vi "实验5 相移键控TX.vi"() -> ()   [LabVIEW 2015]
uses:
  SubVI/SubVI TX Channel Model Params.ctl
  SubVI/SubVI TX HW Aprams.ctl
  <instrlib>/niUSRP/niUSRP Write Tx Data (CDB Cluster).vi
panel:
  out "发送时间":dbl format="%#_4ps"
  out "码元数据量":i32
  in  "设置选项卡":enum32{"硬件设置", "信道设置", "调制设置", "调试显示"}(tab)
  in  "硬件设置":T1={"设备IP地址"="192.168.10.2", "天线"="TX1", "载波频率 (Hz)"=800000000.0, "增益 (dB)"=10.0} {"增益 (dB)" format="%.2f"; "载波频率 (Hz)" format="%.2p"}
  in  "信道模型":T2={"信道模型"="AWGN", "噪声能量 (dB)"=-100.0, "信道响应"=[], "频偏 "=0.0, "延迟 (秒)"=0.0}
  in  "调制设置":T3={"调制方式"="QPSK", "脉冲成形参数 "={"调制方式 "=enum."PSK", "脉冲成形滤波器 "=enum."根升余弦", "滤波器参数"=0.5, "滤波长度 (码元)"=8}, "TX 过采样因子"=4, "TX 采样率"=500000.0} {"TX 采样率" items=["25M"=25000000.0, "20M"=20000000.0, "16.6667M"=16666666.666667, "14.2857M"=14285714.285714, "12.5M"=12500000.0, "11.1111M"=11111111.111111, "10M"=10000000.0, "9.09091M"=9090909.090909, "8.33333M"=8333333.333333, "7.69231M"=7692307.692308, "7.14286M"=7142857.142857, "6.66667M"=6666666.666667, "6.25M"=6250000.0, "5.88235M"=5882352.941176, "5.55556M"=5555555.555556, "5.26316M"=5263157.894737, "5M"=5000000.0, "4.7619M"=4761904.761905, "4.54545M"=4545454.545455, "4.34783M"=4347826.086957, "4.16667M"=4166666.666667, "4M"=4000000.0, "3.84615M"=3846153.846154, "3.7037M"=3703703.703704, "3.57143M"=3571428.571429, "3.44828M"=3448275.862069, "3.33333M"=3333333.333333, "3.22581M"=3225806.451613, "3.125M"=3125000.0, "3.0303M"=3030303.030303, "2.94118M"=2941176.470588, "2.85714M"=2857142.857143, "2.77778M"=2777777.777778, "2.7027M"=2702702.702703, "2.63158M"=2631578.947368, "2.5641M"=2564102.564103, "2.5M"=2500000.0, "2.43902M"=2439024.390244, "2.38095M"=2380952.380952, "2.32558M"=2325581.395349, "2.27273M"=2272727.272727, "2.22222M"=2222222.222222, "2.17391M"=2173913.043478, "2.12766M"=2127659.574468, "2.08333M"=2083333.333333, "2.04082M"=2040816.326531, "2M"=2000000.0, "1.96078M"=1960784.313725, "1.92308M"=1923076.923077, "1.88679M"=1886792.45283, "1.85185M"=1851851.851852, "1.81818M"=1818181.818182, "1.78571M"=1785714.285714, "1.75439M"=1754385.964912, "1.72414M"=1724137.931034, "1.69492M"=1694915.254237, "1.66667M"=1666666.666667, "1.63934M"=1639344.262295, "1.6129M"=1612903.225806, "1.5873M"=1587301.587302, "1.5625M"=1562500.0, "1.53846M"=1538461.538462, "1.51515M"=1515151.515152, "1.49254M"=1492537.313433, "1.47059M"=1470588.235294, "1.44928M"=1449275.362319, "1.42857M"=1428571.428571, "1.40845M"=1408450.704225, "1.38889M"=1388888.888889, "1.36986M"=1369863.013699, "1.35135M"=1351351.351351, "1.33333M"=1333333.333333, "1.31579M"=1315789.473684, "1.2987M"=1298701.298701, "1.28205M"=1282051.282051, "1.26582M"=1265822.78481, "1.25M"=1250000.0, "1.23457M"=1234567.901235, "1.21951M"=1219512.195122, "1.20482M"=1204819.277108, "1.19048M"=1190476.190476, "1.17647M"=1176470.588235, "1.16279M"=1162790.697674, "1.14943M"=1149425.287356, "1.13636M"=1136363.636364, "1.1236M"=1123595.505618, "1.11111M"=1111111.111111, "1.0989M"=1098901.098901, "1.08696M"=1086956.521739, "1.07527M"=1075268.817204, "1.06383M"=1063829.787234, "1.05263M"=1052631.578947, "1.04167M"=1041666.666667, "1.03093M"=1030927.835052, "1.02041M"=1020408.163265, "1.0101M"=1010101.010101, "1M"=1000000.0, "990.099k"=990099.009901, "980.392k"=980392.156863, "970.874k"=970873.786408, "961.538k"=961538.461538, "952.381k"=952380.952381, "943.396k"=943396.226415, "934.579k"=934579.439252, "925.926k"=925925.925926, "917.431k"=917431.192661, "909.091k"=909090.909091, "900.901k"=900900.900901, "892.857k"=892857.142857, "884.956k"=884955.752212, "877.193k"=877192.982456, "869.565k"=869565.217391, "862.069k"=862068.965517, "854.701k"=854700.854701, "847.458k"=847457.627119, "840.336k"=840336.134454, "833.333k"=833333.333333, "826.446k"=826446.280992, "819.672k"=819672.131148, "813.008k"=813008.130081, "806.452k"=806451.612903, "800k"=800000.0, "793.651k"=793650.793651, "787.402k"=787401.574803, "781.25k"=781250.0, "769.231k"=769230.769231, "757.576k"=757575.757576, "746.269k"=746268.656716, "735.294k"=735294.117647, "724.638k"=724637.681159, "714.286k"=714285.714286, "704.225k"=704225.352113, "694.444k"=694444.444444, "684.932k"=684931.506849, "675.676k"=675675.675676, "666.667k"=666666.666667, "657.895k"=657894.736842, "649.351k"=649350.649351, "641.026k"=641025.641026, "632.911k"=632911.392405, "625k"=625000.0, "617.284k"=617283.950617, "609.756k"=609756.097561, "602.41k"=602409.638554, "595.238k"=595238.095238, "588.235k"=588235.294118, "581.395k"=581395.348837, "574.713k"=574712.643678, "568.182k"=568181.818182, "561.798k"=561797.752809, "555.556k"=555555.555556, "549.451k"=549450.549451, "543.478k"=543478.26087, "537.634k"=537634.408602, "531.915k"=531914.893617, "526.316k"=526315.789474, "520.833k"=520833.333333, "515.464k"=515463.917526, "510.204k"=510204.081633, "505.051k"=505050.505051, "500k"=500000.0, "495.05k"=495049.50495, "490.196k"=490196.078431, "485.437k"=485436.893204, "480.769k"=480769.230769, "476.19k"=476190.47619, "471.698k"=471698.113208, "467.29k"=467289.719626, "462.963k"=462962.962963, "458.716k"=458715.59633, "454.545k"=454545.454545, "450.45k"=450450.45045, "446.429k"=446428.571429, "442.478k"=442477.876106, "438.596k"=438596.491228, "434.783k"=434782.608696, "431.034k"=431034.482759, "427.35k"=427350.42735, "423.729k"=423728.813559, "420.168k"=420168.067227, "416.667k"=416666.666667, "413.223k"=413223.140496, "409.836k"=409836.065574, "406.504k"=406504.065041, "403.226k"=403225.806452, "400k"=400000.0, "396.825k"=396825.396825, "393.701k"=393700.787402, "390.625k"=390625.0, "384.615k"=384615.384615, "378.788k"=378787.878788, "373.134k"=373134.328358, "367.647k"=367647.058824, "362.319k"=362318.84058, "357.143k"=357142.857143, "352.113k"=352112.676056, "347.222k"=347222.222222, "342.466k"=342465.753425, "337.838k"=337837.837838, "333.333k"=333333.333333, "328.947k"=328947.368421, "324.675k"=324675.324675, "320.513k"=320512.820513, "316.456k"=316455.696203, "312.5k"=312500.0, "308.642k"=308641.975309, "304.878k"=304878.04878, "301.205k"=301204.819277, "297.619k"=297619.047619, "294.118k"=294117.647059, "290.698k"=290697.674419, "287.356k"=287356.321839, "284.091k"=284090.909091, "280.899k"=280898.876404, "277.778k"=277777.777778, "274.725k"=274725.274725, "271.739k"=271739.130435, "268.817k"=268817.204301, "265.957k"=265957.446809, "263.158k"=263157.894737, "260.417k"=260416.666667, "257.732k"=257731.958763, "255.102k"=255102.040816, "252.525k"=252525.252525, "250k"=250000.0, "247.525k"=247524.752475, "245.098k"=245098.039216, "242.718k"=242718.446602, "240.385k"=240384.615385, "238.095k"=238095.238095, "235.849k"=235849.056604, "233.645k"=233644.859813, "231.481k"=231481.481481, "229.358k"=229357.798165, "227.273k"=227272.727273, "225.225k"=225225.225225, "223.214k"=223214.285714, "221.239k"=221238.938053, "219.298k"=219298.245614, "217.391k"=217391.304348, "215.517k"=215517.241379, "213.675k"=213675.213675, "211.864k"=211864.40678, "210.084k"=210084.033613, "208.333k"=208333.333333, "206.612k"=206611.570248, "204.918k"=204918.032787, "203.252k"=203252.03252, "201.613k"=201612.903226, "200k"=200000.0, "198.413k"=198412.698413, "196.85k"=196850.393701, "195.312k"=195312.5]}
  out "载波频率":dbl=1200000000.0 format="%#_6p"
  out "强制增益(dB)":dbl=1000000.0 format="%#_6f"
  out "打包持续时间(s)":dbl=0.021552 min=50000000.0 max=100000000.0 step=50000000.0 format="%#_6p"
  out "码元速率(Hz)":dbl=250000.0 min=50000000.0 max=100000000.0 step=50000000.0 format="%#_6p"
  out "实际延迟(s)":dbl
  out "强制 IQ 速率":dbl=10.0 format="%#_6p"
  in  "发送文本":string="    What is success？  \n　　To laugh often and love much；\n　　To win the respect of intelligent people  \n　　And the affection of children；  \n　　To earn the approbation of honest critics  \n　　And endure the betrayal of false friends；  \n　　To appreciate beauty；  \n　　To find the best in others；  \n　　To give oneself；  \n　　To leave the world a little better，  \n    Whether by a healthy child，  \n    A garden patch，  \n　　Or a redeemed social condition；  \n　　To have played and laughed with enthusiasm  \n　　And sung with exultation；  \n　　To know even one life has breathed easier，  \n　　Because you have lived……  \n　　This is to have succeeded.\n"
  in  "图形选项卡":enum32{"信号星座图", "信号眼图", "信号IQ波形"}(tab)=enum."信号IQ波形"
  out "星座图":cluster{dbl[], dbl[]}(graph)
  out "眼图":cluster{"t0":dbl, "dt":dbl, "Y":dbl[]}[](graph)
  out "输出IQ波形":cluster{"t0":dbl, "dt":dbl, "Y":dbl[]}(graph)={"t0"=0.0, "dt"=1e-06, "Y"=[]}
  out "传输状态":bool=TRUE
  in  "停止":bool
  out "当前状态":string="正在传输……"
  # "实验5 相移键控TX"
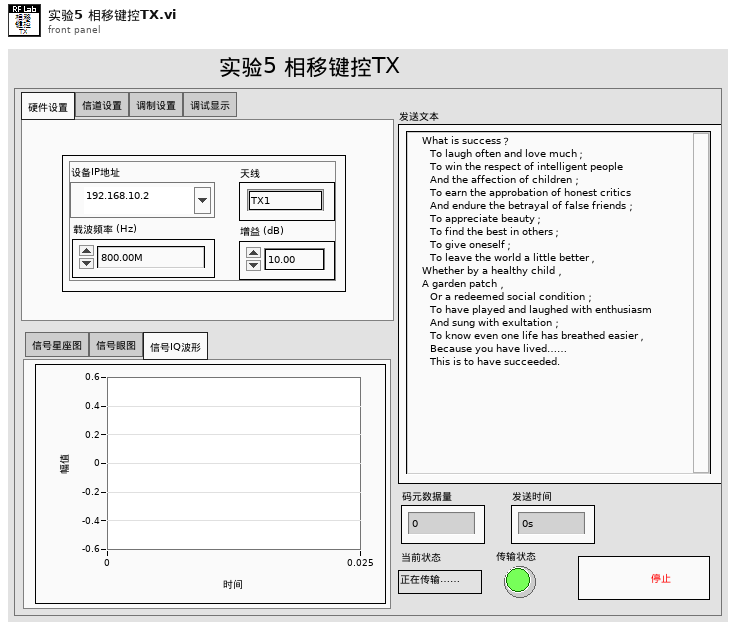
[diagram p1: front panel]
types:
  T1 = typedef "SubVI TX HW Aprams.ctl" = cluster{"设备IP地址":refnum<k15>, "天线":string, "载波频率 (Hz)":dbl, "增益 (dB)":dbl}
  T2 = typedef "SubVI TX Channel Model Params.ctl" = cluster{"信道模型":string, "噪声能量 (dB)":dbl, "信道响应":cdb[], "频偏 ":dbl, "延迟 (秒)":dbl}
  T3 = cluster{"调制方式":string, "脉冲成形参数 ":cluster{"调制方式 ":enum16{"FSK", "PSK", "QAM", "MSK", "PAM", "ASK"}, "脉冲成形滤波器 ":enum16{"无", "升余弦", "根升余弦", "高斯"}, "滤波器参数":dbl, "滤波长度 (码元)":i32}, "TX 过采样因子":i32, "TX 采样率":dbl}
  T4 = typedef "SubVI TX Modulation Params .ctl" = cluster{"调制方式":string, "脉冲成形参数 ":cluster{"调制方式 ":enum16{"FSK", "PSK", "QAM", "MSK", "PAM", "ASK"}, "脉冲成形滤波器 ":enum16{"无", "升余弦", "根升余弦", "高斯"}, "滤波器参数":dbl, "滤波长度 (码元)":i32}, "RX 过采样因子":i32, "RX 采样率":dbl}
  T5 = cluster{"coerced gain":dbl, "coerced carrier frequency":dbl, "coerced IQ rate":dbl}
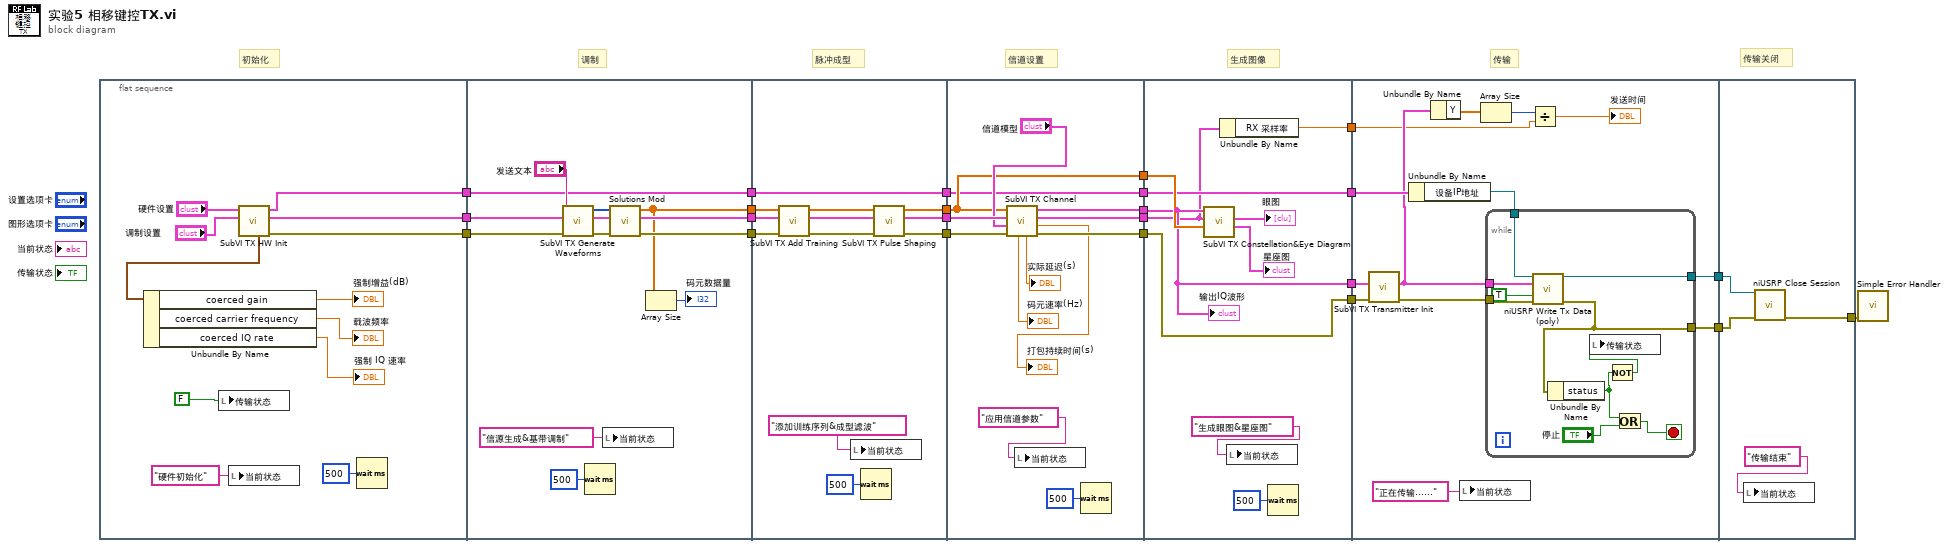
[diagram p0: block diagram]
diagram:
  # "传输关闭"
  # "传输"
  # "生成图像"
  # "信道设置"
  # "脉冲成型"
  # "调制"
  # "初始化"
  n1 = flat-sequence {
    tunnel: [w34] -> w23
    tunnel: [w33] -> w22
    tunnel: [w29] -> w21
    tunnel: w23 -> [w41]
    tunnel: w22 -> [w48]
    tunnel: w21 -> [w46]
    tunnel: [w36] -> w20
    tunnel: [w43] -> w19
    tunnel: [w42] -> w18
    tunnel: [w41] -> w17
    tunnel: w20 -> [w60]
    tunnel: w19 -> [w59]
    tunnel: w18 -> [w58]
    tunnel: w17 -> [w49]
    tunnel: [w52] -> w16
    tunnel: [w51] -> w15
    tunnel: [w50] -> w14
    tunnel: [w49] -> w8
    tunnel: w16 -> [w66]
    tunnel: w15 -> [w73]
    tunnel: w14 -> [w72]
    tunnel: [w70] -> w13
    tunnel: [w69] -> w12
    tunnel: [w68] -> w11
    tunnel: [w66] -> w10
    tunnel: [w61] -> w9
    tunnel: w8 -> [w61]
    tunnel: w13 -> [w78]
    tunnel: w12 -> [w75]
    tunnel: w11 -> [w77]
    tunnel: w10 -> [w83]
    tunnel: w9 -> [w79]
    tunnel: [w79] -> w7
    tunnel: [w78] -> w6
    tunnel: [w77] -> w5
    tunnel: [w74] -> w1
    tunnel: w7 -> [w95]
    tunnel: w6 -> [w96]
    tunnel: w5 -> [w90]
    tunnel: [w93] -> w4
    tunnel: [w92] -> w3
    tunnel: w1 -> [w85]
    tunnel: w4 -> [w109]
    tunnel: w3 -> [w110]
    tunnel: [w108] -> w2
    frame #0 {
      n2 = local write "传输状态"(FALSE ("传输？")) -> ()
      n3 = local write "当前状态"("硬件初始化" ("当前状态")) -> ()
      n4 = call "SubVI TX HW Init.vi"("调制设置"="调制设置", "硬件设置"="硬件设置") -> ("错误输出"=w29:errorcluster, "调制设置"=w33:T4, "硬件设置"=w34:T1, "硬件参数"=w27:T5)  [unwired: 6 in]
      n5 = Unbundle By Name(w27) -> ("coerced gain"=→"强制增益(dB)":dbl, "coerced carrier frequency"=→"载波频率":dbl, "coerced IQ rate"=→"强制 IQ 速率":dbl)
      n6 = Wait (ms)(milliseconds to wait=u32 500 ("等待时间（毫秒）")) -> ()  [unwired: 1 out]
    }
    frame #1 {
      n7 = call "SubVI TX Generate Waveforms.vi"("错误输入"=w46, "文本"="发送文本", "调制设置"=w48) -> ("错误输出"=w44:errorcluster, "调制设置"=w45:T4, "输出位序列"=w38:i8[])  [unwired: 4 in, 2 out]
      n8 = Wait (ms)(milliseconds to wait=u32 500 ("等待时间（毫秒）")) -> ()  [unwired: 1 out]
      n9 = local write "当前状态"("信源生成&基带调制" ("当前状态")) -> ()
      n10 = call "Solutions Mod.vi"("错误输入"=w44, "调制设置"=w45, "输入比特流"=w38) -> ("错误输出"=w42:errorcluster, "调制设置"=w43:T4, "输出符号"=w36:cdb[])  [unwired: 6 in]
      n11 = Array Size(array=w36) -> (size(s)=→"码元数据量":i32)
    }
    frame #2 {
      n12 = call "SubVI TX Add Training .vi"("错误输入"=w58, "调制设置"=w59, "输入"=w60) -> ("错误输出"=w55:errorcluster, "调制设置"=w56:T4, "输出"=w57:cdb[])  [unwired: 5 in, 1 out]
      n13 = local write "当前状态"("添加训练序列&成型滤波" ("当前状态")) -> ()
      n14 = Wait (ms)(milliseconds to wait=u32 500 ("等待时间（毫秒）")) -> ()  [unwired: 1 out]
      n15 = call "SubVI TX Pulse Shaping .vi"("错误输入"=w55, "调制设置"=w56, "输入"=w57) -> ("错误输出"=w50:errorcluster, "调制设置"=w51:T4, "输出"=w52:cdb[])  [unwired: 6 in]
    }
    frame #3 {
      n16 = call "SubVI TX Channel.vi"("错误输入"=w72, "通道型号参数"="信道模型", "调制设置"=w73, "输入波形"=w66) -> ("错误输出"=w68:errorcluster, "分组持续时间(s)"=→"打包持续时间(s)":dbl, "调制设置"=w69:T4, "输出复杂波形"=w70:cluster{"t0":dbl, "dt":dbl, "Y":cdb[]}, "实际延迟(s)"=→"实际延迟(s)":dbl, "符号率(Hz)"=→"码元速率(Hz)":dbl)  [unwired: 2 in]
      n17 = local write "当前状态"("应用信道参数" ("当前状态")) -> ()
      n18 = Wait (ms)(milliseconds to wait=u32 500 ("等待时间（毫秒）")) -> ()  [unwired: 1 out]
    }
    frame #4 {
      n19 = call "SubVI TX Constellation&Eye Diagram.vi"("输入符号"=w83, "调制设置"=w75, "复杂波形"=w78) -> ("传输的星座图"=→"星座图":cluster{dbl[], dbl[]}, "眼图"=→"眼图":cluster{"t0":dbl, "dt":dbl, "Y":dbl[]}[])  [unwired: 5 in, 2 out]
      n20 = Unbundle By Name(w75) -> ("RX 采样率"=w74:dbl)
      n21 = local write "当前状态"("生成眼图&星座图" ("当前状态")) -> ()
      n22 = Wait (ms)(milliseconds to wait=u32 500 ("等待时间（毫秒）")) -> ()  [unwired: 1 out]
      "输出IQ波形" <- w78
    }
    frame #5 {
      n23 = call "SubVI TX Transmitter Init.vi"("错误输入"=w90, "IQ数据"=w96) -> ("错误输出"=w89:errorcluster, "缩放和填充IQ数据"=w88:cluster{"t0":dbl, "dt":dbl, "Y":cdb[]})  [unwired: 8 in]
      n24 = Unbundle By Name(w95) -> ("设备IP地址"=w94:refnum<k15>)
      n25 = Unbundle By Name(w88) -> ("Y"=w87:cdb[])
      n26 = local write "当前状态"("正在传输……" ("当前状态")) -> ()
      n27 = Array Size(array=w87) -> (size(s)=w86:i32)
      n28 = while {
        tunnel: w88 -> [w105]
        tunnel: w89 -> [w104]
        tunnel: w94 -> [w106]
        tunnel: [w103] -> w93
        tunnel: [w101] -> w92
        stop <- w99 stop-if-true
        n29 = call-poly <instrlib>:"niUSRP Write Tx Data (poly).vi"("session handle"=w106, "data"=w105, "end of data?"=TRUE, "error in (no error)"=w104) -> ("session handle out"=w101:refnum<k15>, "error out"=w103:errorcluster)  [unwired: 10 in]
        n30 = Unbundle By Name(w103) -> ("status"=w97:bool)
        n31 = Not(x=w97) -> (.not. x?=w98:bool)
        n32 = local write "传输状态"(w98) -> ()
        n33 = Or(x=w97, y="停止") -> (x .or. y?=w99:bool)
      }
      n34 = Divide(x=w86, y=w85) -> (x/y=→"发送时间":dbl)
    }
    frame #6 {
      n35 = local write "当前状态"("传输结束" ("当前状态")) -> ()
      n36 = call <instrlib>:"niUSRP Close Session.vi"("session handle"=w110, "error in (no error)"=w109) -> ("error out"=w108:errorcluster)  [unwired: 13 in]
    }
  }
  n37 = call <vilib>:"Simple Error Handler.vi"("error in (no error)"=w2) -> ()  [unwired: 4 in, 5 out]
